vi "Actor Core.vi"(8 "error in":errorcluster caption="错误输入", 11 "P3AT in":refnum<class "RemoteP3AT.lvclass"> caption="操作者输入") -> (0 "error out":errorcluster caption="错误输出", 3 "Actor out":refnum<class "Actor.lvclass"> caption="操作者输出")   [LabVIEW 2014, in "RemoteP3AT.lvlib" / "RemoteP3AT.lvclass"]
doc: "(<B>文件名</B>：Actor Framework.lvlib:Actor.lvclass:Actor Core.vi)\n\n接收发送至操作者的消息，响应消息并处理可能导致操作者关闭的错误。\n\n子孙类重写该VI，使操作者完成特定的任务。使用调用父方法节点实现重写。"
uses:
  RemoteP3AT.lvclass
  <vilib>/ActorFramework/Actor/Actor.lvclass
  ctl/Point.ctl
  ctl/P3AT_Panel.ctl
  <userlib>/ROS for LabVIEW Software/ROS/Code/Console/Servers/ServerSubs/TopicDef.ctl
  <userlib>/ROS for LabVIEW Software/ROS/Code/SubVIs/_ROSDirection.ctl
  RemoteP3AT.lvclass/RemoteP3AT.ctl
  <vilib>/ActorFramework/Actor/Actor.lvclass/Actor.ctl
  <vilib>/ActorFramework/Message Enqueuer/Message Enqueuer.lvclass/Message Enqueuer.ctl
  <vilib>/ActorFramework/Message Enqueuer/Enqueue.vi
  Global_var/Global_var.vi
  <vilib>/ActorFramework/Message Priority Queue/Priority Enqueue.vi
  Wrapper_lib/zsActor/ActorWrapper.lvclass
panel:
  out "P3AT_Ini_Pose":T1
  out "P3AT_Panel":T2={"max_vel"=0.49056603773584906, "max_rot"=0.5094339622641509, "Control_Mode"=enum."Joy"} {"max_rot" scale=0.0..1.0; "max_vel" scale=0.0..1.0}
  out "vel_cal":cluster{"rot_z":dbl, "lin_x":dbl}
  out "local_goal":T3
  in  "停止信号":bool
  # "P3AT_Panel 此处不起作用"
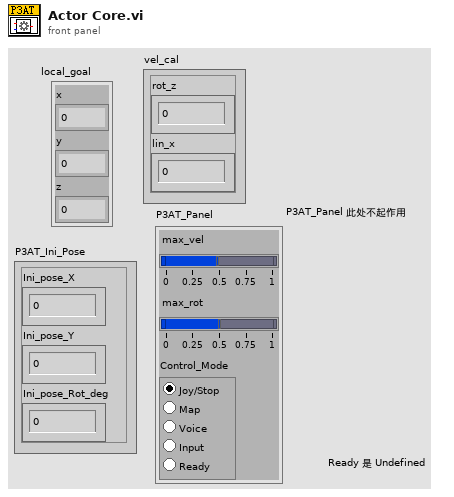
[diagram p1: front panel]
types:
  T1 = cluster{"Ini_pose_X":dbl, "Ini_pose_Y":dbl, "Ini_pose_Rot_deg":dbl}
  T2 = typedef "P3AT_Panel.ctl" = cluster{"max_vel":dbl, "max_rot":dbl, "Control_Mode":enum32{"Joy", "Map", "Voice", "Input", "Undefined"}}
  T3 = typedef "Point.ctl" = cluster{"x":dbl, "y":dbl, "z":dbl}
  T4 = typedef "TopicDef.ctl" = cluster{"Topic":string, "Type":string, "Action":T5, "Update (ms)":u16, "queue size":u16}
  T5 = typedef "_ROSDirection.ctl" = enum16{"Node", "Publisher", "Subscriber", "ServiceClient", "ServiceProvider"}
  T6 = typedef "_ROSControl.ctl" = cluster{"topic port":u16, "Node":string, "topic":string, "type":string, "node port":u16, "error ":errorcluster, "Direction":T5, "Update (ms)":u16, "FIFO size":u16}
  T7 = enum32{"Joy", "Map", "Voice", "Input", "Undefined"}
  T8 = typedef "P3AT_Current.ctl" = cluster{"max_vel":dbl, "max_rot":dbl, "now_pose_X":dbl, "now_pose_Y":dbl, "now_pose_Rot_deg":dbl, "Control_Mode":enum32{"Joy", "Map", "Voice", "Input", "Undefined"}}
  T9 = cluster{"now_pose_X":dbl, "now_pose_Y":dbl, "now_pose_Rot_deg":dbl}
  T10 = typedef "Robot_Position.ctl" = cluster{"global x":dbl, "global y":dbl, "global z":dbl, "global_rot":dbl, " floor NO.":dbl}
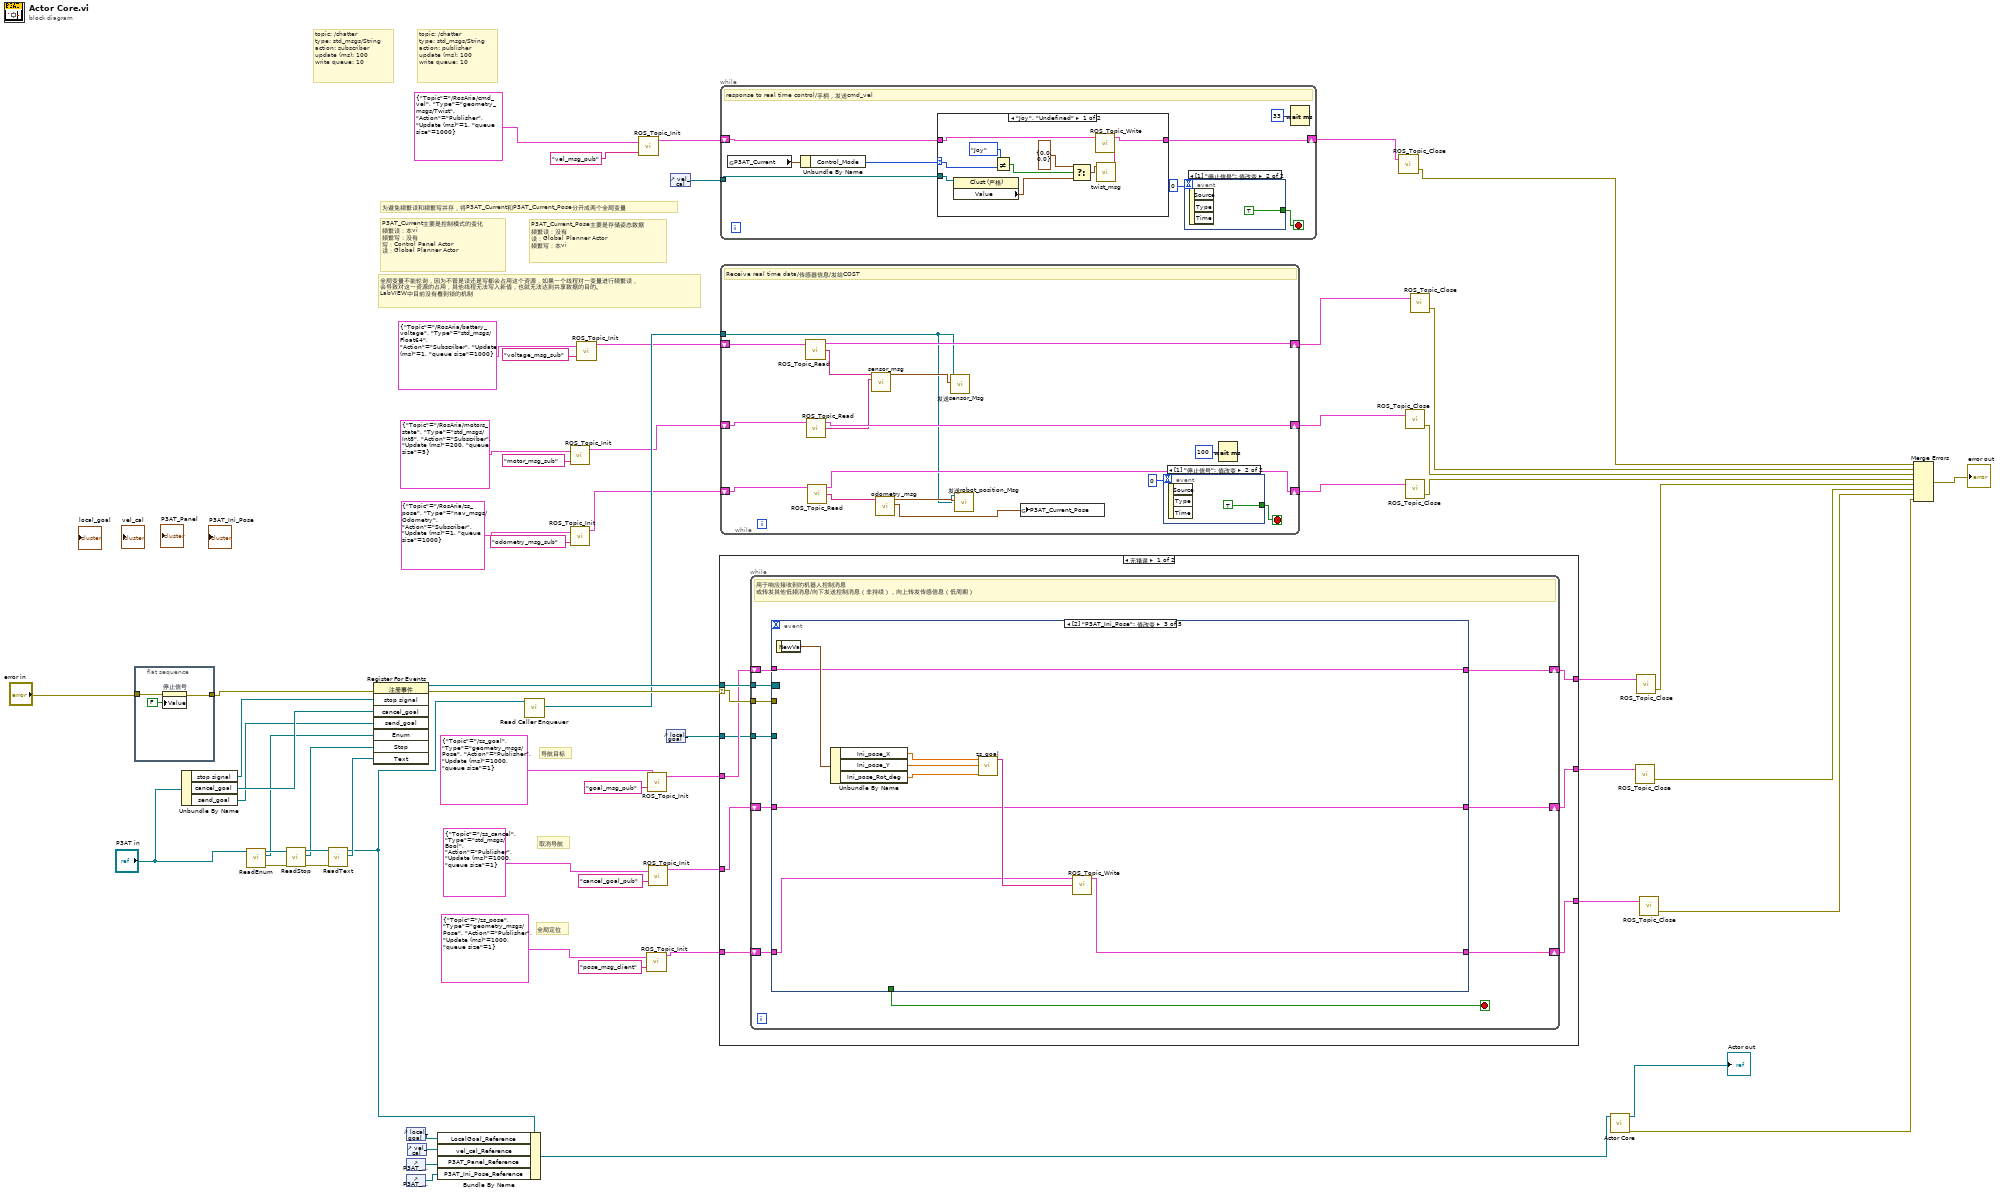
[diagram p0: block diagram]
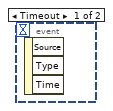
[diagram p3: hidden frame]
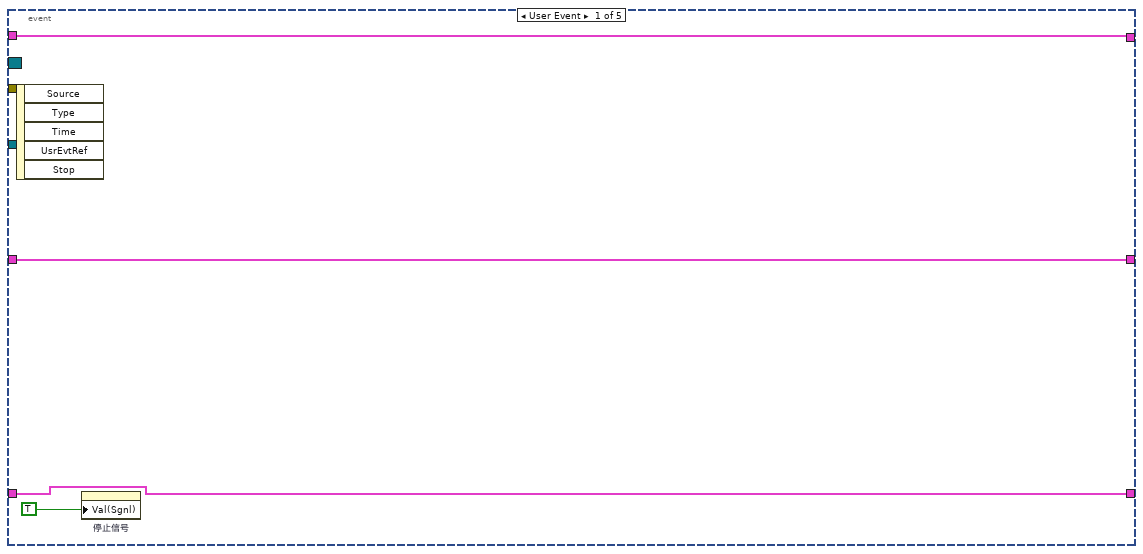
[diagram p4: hidden frame]
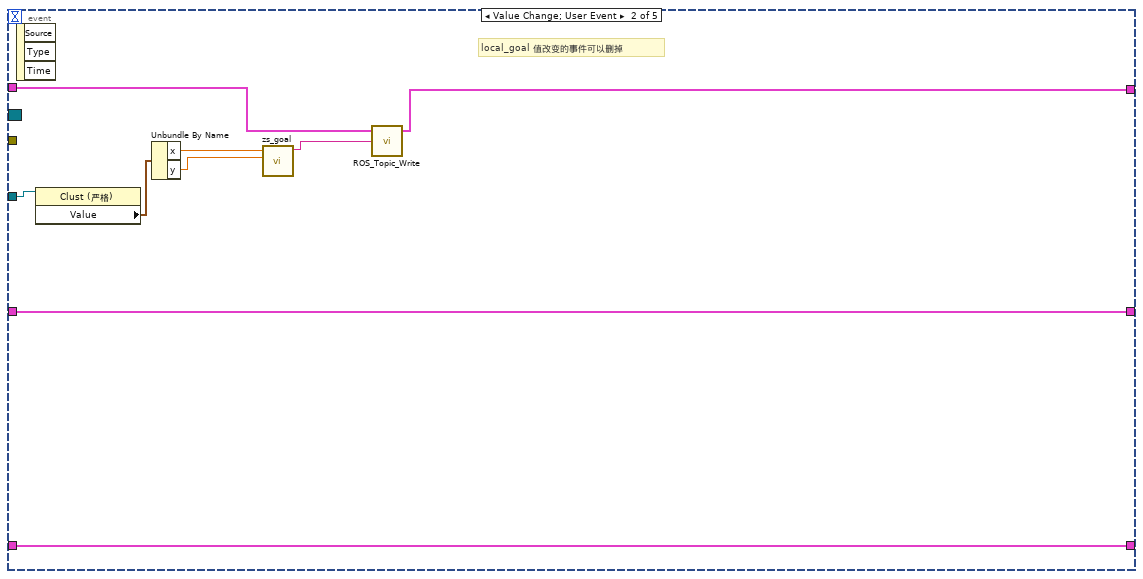
[diagram p5: hidden frame]
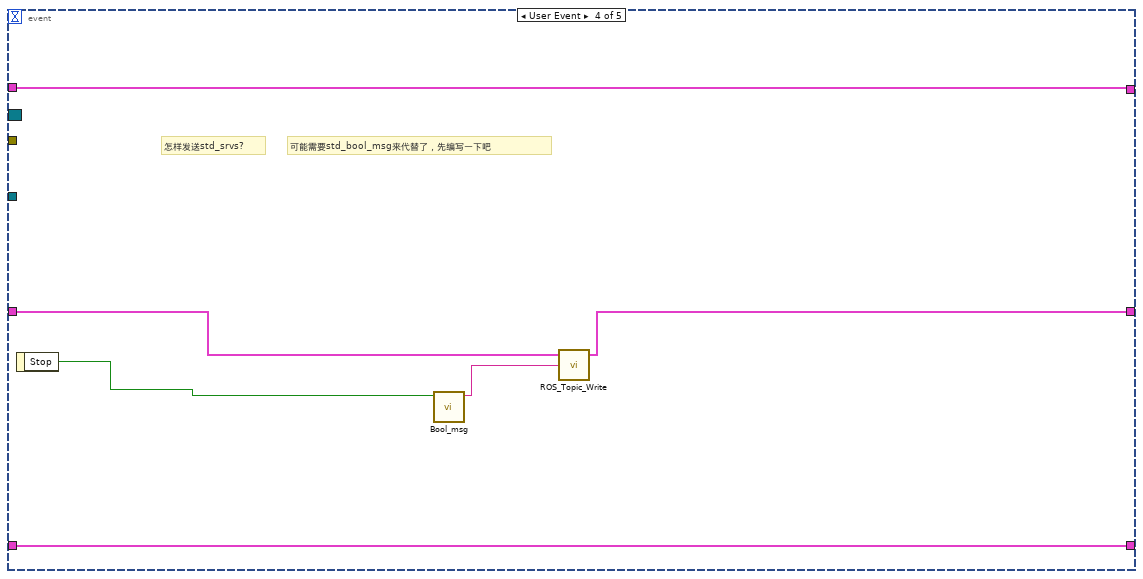
[diagram p6: hidden frame]
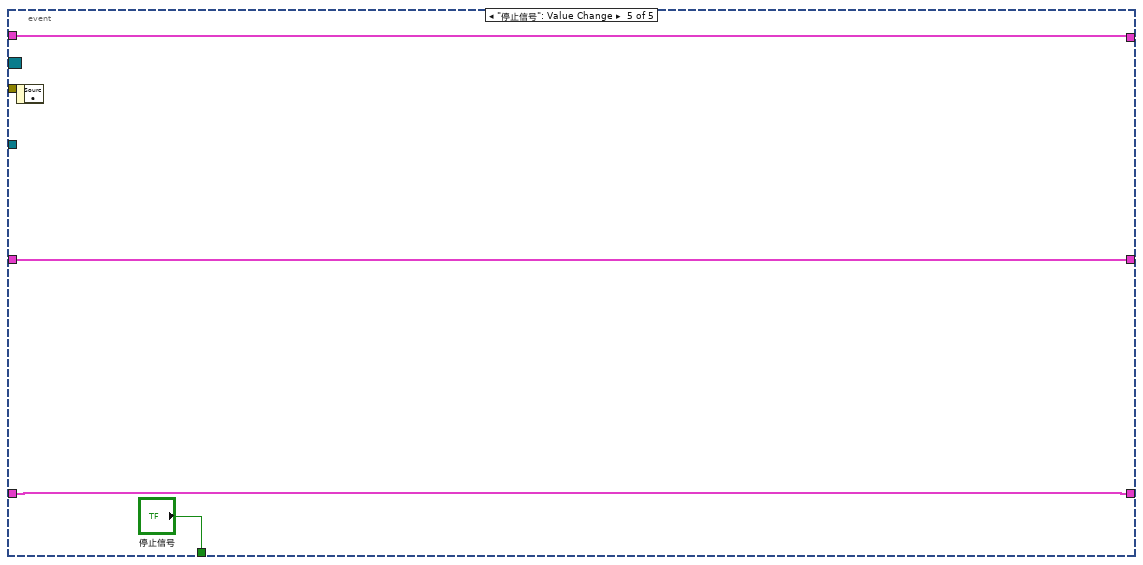
[diagram p7: hidden frame]
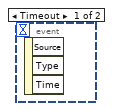
[diagram p9: hidden frame]
diagram:
  # "全局变量不能轮询，因为不管是读还是写都会占用这个资源，如果一个线程对一变量进行频繁读，\n会导致对这一资源的占用，其他线程无法写入新值，也就无法达到共享数据的目的。\nLabVIEW中目前没有看到锁的机制"
  # "全局定位"
  # "P3AT_Current_Pose主要是存储姿态数据\n频繁读：没有\n读：Global Planner Actor\n频繁写：本vi"
  # "P3AT_Current主要是控制模式的变化\n频繁读：本vi\n频繁写：没有\n写：Control Panel Actor\n读：Global Planner Actor"
  # "为避免频繁读和频繁写并存，将P3AT_Current和P3AT_Current_Pose分开成两个全局变量"
  # "导航目标"
  # "取消导航"
  # "topic: /chatter\ntype: std_msgs/String\naction: subscriber\nupdate (ms): 100\nwrite queue: 10"
  # "topic: /chatter\ntype: std_msgs/String\naction: publisher\nupdate (ms): 100\nwrite queue: 10"
  n1 = flat-sequence {
    tunnel: [w64] -> w58
    tunnel: "error in" -> [w63]
    frame #0 {
      n2 = property on="停止信号" class="Bool (严格)"(error in=w63, "Value"=FALSE ("停止信号")) -> (error out=w64:errorcluster)  [unwired: 1 in, 1 out]
    }
  }
  n3 = Unbundle By Name("P3AT in") -> ("stop signal"=w57:refnum<user-event>, "cancel_goal"=w56:refnum<user-event>, "send_goal"=w1:refnum<user-event>)
  n4 = call-dynamic "ReadEnum.vi"("zsActor输入"="P3AT in") -> ("error out"=w53:errorcluster, "Enum"=w50:refnum<user-event>, "zsActor输出"=w55:refnum<class "RemoteP3AT.lvclass">)  [unwired: 8 in]
  n5 = call-dynamic "ReadStop.vi"("error in (no error)"=w53, "zsActor输入"=w55) -> ("error out"=w52:errorcluster, "Stop"=w49:refnum<user-event>, "zsActor输出"=w54:refnum<class "RemoteP3AT.lvclass">)  [unwired: 7 in]
  n6 = call-dynamic "ReadText.vi"("error in (no error)"=w52, "zsActor输入"=w54) -> ("Text"=w48:refnum<user-event>, "zsActor输出"=w19:refnum<class "RemoteP3AT.lvclass">)  [unwired: 7 in, 1 out]
  n7 = register-events(error in=w58, w57, w56, w1, w50, w49, w48) -> (reference out=w60:refnum<event-registration>, error out=w61:errorcluster)  [unwired: 1 in]
  n8 = control-ref of="P3AT_Panel"() -> (w10:refnum<vi>)
  n9 = control-ref of="local_goal"() -> (w17:refnum<vi>)
  n10 = control-ref of="P3AT_Ini_Pose"() -> (w3:refnum<vi>)
  n11 = control-ref of="vel_cal"() -> (w12:refnum<vi>)
  n12 = Bundle By Name(cluster=w19, "LocalGoal_Reference"=w17, "vel_cal_Reference"=w12, "P3AT_Panel_Reference"=w10, "P3AT_Ini_Pose_Reference"=w3) -> (w18:refnum<class "RemoteP3AT.lvclass">)
  n13 = call <vilib>:"Read Caller Enqueuer.vi"("Actor"=w19) -> ("Caller Enqueuer"=w47:refnum<class "Message Enqueuer.lvclass">)  [unwired: 10 in]
  n14 = call <userlib>:"ROS_Topic_Init.vi"("Definitions"=T4 {"Topic"="/RosAria/motors_state", "Type"="std_msgs/Int8", "Action"=enum."Subscriber", "Update (ms)"=200, "queue size"=5}, "node"="motor_msg_sub") -> ("ROS out"=w28:T6)  [unwired: 1 in, 1 out]
  n15 = call <userlib>:"ROS_Topic_Init.vi"("Definitions"=T4 {"Topic"="/RosAria/zs_pose", "Type"="nav_msgs/Odometry", "Action"=enum."Subscriber", "Update (ms)"=1, "queue size"=1000}, "node"="odometry_msg_sub") -> ("ROS out"=w24:T6)  [unwired: 1 in, 1 out]
  n16 = call <userlib>:"ROS_Topic_Init.vi"("Definitions"=T4 {"Topic"="/RosAria/battery_voltage", "Type"="std_msgs/Float64", "Action"=enum."Subscriber", "Update (ms)"=1, "queue size"=1000}, "node"="voltage_msg_sub") -> ("ROS out"=w30:T6)  [unwired: 1 in, 1 out]
  n17 = call <userlib>:"ROS_Topic_Init.vi"("Definitions"=T4 {"Topic"="/RosAria/cmd_vel", "Type"="geometry_msgs/Twist", "Action"=enum."Publisher", "Update (ms)"=1, "queue size"=1000}, "node"="vel_msg_pub") -> ("ROS out"=w31:T6)  [unwired: 1 in, 1 out]
  n18 = call <userlib>:"ROS_Topic_Init.vi"("Definitions"=T4 {"Topic"="/zs_pose", "Type"="geometry_msgs/Pose", "Action"=enum."Publisher", "Update (ms)"=1000, "queue size"=1}, "node"="pose_msg_client") -> ("ROS out"=w4:T6)  [unwired: 1 in, 1 out]
  n19 = call <userlib>:"ROS_Topic_Init.vi"("Definitions"=T4 {"Topic"="/zs_goal", "Type"="geometry_msgs/Pose", "Action"=enum."Publisher", "Update (ms)"=1000, "queue size"=1}, "node"="goal_msg_pub") -> ("ROS out"=w16:T6)  [unwired: 1 in, 1 out]
  n20 = call <userlib>:"ROS_Topic_Init.vi"("Definitions"=T4 {"Topic"="/zs_cancel", "Type"="std_msgs/Bool", "Action"=enum."Publisher", "Update (ms)"=1000, "queue size"=1}, "node"="cancel_goal_pub") -> ("ROS out"=w15:T6)  [unwired: 1 in, 1 out]
  n21 = control-ref of="local_goal"() -> (w9:refnum<vi>)
  n22 = control-ref of="vel_cal"() -> (w11:refnum<vi>)
  n23 = case shown="无错误" w61 {
    selector: w61 -> [w73 _]
    tunnel: w60 -> [w74 _]
    tunnel: w16 -> [w72 w119]
    tunnel: w15 -> [w71 w118]
    tunnel: [w70 w119] -> w14
    tunnel: [w69 w118] -> w13
    tunnel: w9 -> [w68 _]
    tunnel: w4 -> [w67 w117]
    tunnel: [w66 w117] -> w2
    frame No Error {
      n24 = while {
        tunnel: w74 -> [w84]
        tunnel: w73 -> [w82]
        shift-right: [w81] -> w70
        shift-left: w72 -> [w80]
        shift-right: [w78] -> w69
        shift-left: w71 -> [w79]
        tunnel: w68 -> [w77]
        shift-right: [w75] -> w66
        shift-left: w67 -> [w76]
        stop <- w83 stop-if-true
        # "用于响应接收到的机器人控制消息\n或转发其他低频消息/向下发送控制消息（非持续），向上转发传感信息（低周期）"
        n25 = event shown="[2] \"P3AT_Ini_Pose\": 值改变" {
          selector: w84 -> [_ _ _ _ _]
          dyn-events: _ -> [_ _ _ _ _]
          timeout: _ -> [_ _ _ _ _]
          tunnel: [_ _ _ _ "停止信号"] -> w83
          tunnel: w82 -> [_ _ _ _ _]
          tunnel: w80 -> [w87 w95 w98 w110 w115]
          tunnel: [w87 w93 w98 w110 w115] -> w81
          tunnel: w79 -> [w86 w92 w99 w112 w114]
          tunnel: [w86 w92 w99 w111 w114] -> w78
          tunnel: w77 -> [_ w91 _ _ _]
          tunnel: w76 -> [w85 w89 w101 w109 w113]
          tunnel: [w85 w89 w100 w109 w113] -> w75
          event User Event {
            n26 = event-data() -> ()  [unwired: 1 in, 5 out]
            n27 = property on="停止信号" class="Bool (严格)"("Val(Sgnl)"=TRUE ("值(信号)")) -> ()  [unwired: 2 in, 2 out]
          }
          event Value Change; User Event {
            # "local_goal 值改变的事件可以删掉"
            n28 = event-data() -> ()  [unwired: 1 in, 3 out]
            n29 = property class="Clust (严格)"(reference=w91) -> ("Value"=w90:T3)  [unwired: 1 in, 2 out]
            n30 = Unbundle By Name(w90) -> ("x"=w97:dbl, "y"=w96:dbl)
            n31 = call "zs_goal.vi"("Point.y"=w96, "Point.x"=w97) -> ("msg out"=w94:string)  [unwired: 9 in]
            n32 = call <userlib>:"ROS_Topic_Write.vi"("Msg in"=w94, "ROS in"=w95) -> ("ROS out"=w93:T6)  [unwired: 2 in, 1 out]
          }
          event "P3AT_Ini_Pose": Value Change {
            n33 = event-data() -> ("NewVal"=w106:T1)  [unwired: 1 in]
            n34 = Unbundle By Name(w106) -> ("Ini_pose_X"=w105:dbl, "Ini_pose_Y"=w104:dbl, "Ini_pose_Rot_deg"=w103:dbl)
            n35 = call "zs_goal.vi"("Yaw (z)"=w103, "Point.y"=w104, "Point.x"=w105) -> ("msg out"=w102:string)  [unwired: 8 in]
            n36 = call <userlib>:"ROS_Topic_Write.vi"("Msg in"=w102, "ROS in"=w101) -> ("ROS out"=w100:T6)  [unwired: 2 in, 1 out]
          }
          event User Event {
            # "可能需要std_bool_msg来代替了，先编写一下吧"
            # "怎样发送std_srvs?"
            n37 = event-data() -> ("Stop"=w107:bool)  [unwired: 1 in]
            n38 = call "Bool_msg.vi"("Boolean"=w107) -> ("msg out"=w108:string)  [unwired: 10 in]
            n39 = call <userlib>:"ROS_Topic_Write.vi"("Msg in"=w108, "ROS in"=w112) -> ("ROS out"=w111:T6)  [unwired: 2 in, 1 out]
          }
          event "停止信号": Value Change {
            n40 = event-data() -> ()  [unwired: 1 in, 1 out]
          }
        }
      }
    }
    frame Error {
    }
  }
  n41 = while {
    shift-right: [w123] -> w32
    shift-left: w31 -> [w124]
    tunnel: w11 -> [w122]
    stop <- w126 stop-if-true
    # "response to real time control/手柄，发送cmd_vel"
    n42 = global read "Global_var.vi" "P3AT_Current"() -> (w120:T8)
    n43 = Unbundle By Name(w120) -> ("Control_Mode"=w121:T7)
    n44 = case shown="\"Joy\", \"Undefined\"" w121 {
      selector: w121 -> [w132 _]
      tunnel: w124 -> [w137 w138]
      tunnel: [w136 w138] -> w123
      tunnel: w122 -> [w135 _]
      frame "Joy", "Undefined" {
        n45 = property class="Clust (严格)"(reference=w135) -> ("Value"=w130:cluster{"rot_z":dbl, "lin_x":dbl})  [unwired: 1 in, 2 out]
        n46 = Not Equal?(x=T7."Joy" ("Control_Mode"), y=w132) -> (x != y?=w131:bool)
        n47 = Select(t=cluster{"rot_z":dbl, "lin_x":dbl} {"rot_z"=0.0, "lin_x"=0.0} ("值"), s=w131, f=w130) -> (s? t:f=w128:cluster{"rot_z":dbl, "lin_x":dbl})
        n48 = call "twist_msg.vi"("vel_cal"=w128) -> ("msg out"=w134:string)  [unwired: 10 in]
        n49 = call <userlib>:"ROS_Topic_Write.vi"("Msg in"=w134, "ROS in"=w137) -> ("ROS out"=w136:T6)  [unwired: 2 in, 1 out]
      }
      frame "Map".."Input", Default {
      }
    }
    n50 = event shown="[1] \"停止信号\": 值改变" {
      selector: _ -> [_ _]
      dyn-events: _ -> [_ _]
      timeout: 0 -> [_ _]
      tunnel: [_ TRUE] -> w126
      event Timeout {
        n51 = event-data() -> ()  [unwired: 1 in, 3 out]
      }
      event "停止信号": Value Change {
        n52 = event-data() -> ()  [unwired: 1 in, 3 out]
      }
    }
    n53 = Wait (ms)(milliseconds to wait=u32 33 ("等待时间（毫秒）")) -> ()  [unwired: 1 out]
  }
  n54 = while {
    tunnel: w47 -> [w141]
    shift-right: [w151] -> w29
    shift-left: w30 -> [w152]
    shift-right: [w149] -> w27
    shift-left: w28 -> [w150]
    shift-right: [w147] -> w23
    shift-left: w24 -> [w148]
    stop <- w154 stop-if-true
    # "Receive real time data/传感器信息/发给COST"
    n55 = call <userlib>:"ROS_Topic_Read.vi"("ROS in"=w152) -> ("Reply"=w146:string, "ROS out"=w151:T6)  [unwired: 2 in, 1 out]
    n56 = call <userlib>:"ROS_Topic_Read.vi"("ROS in"=w150) -> ("Reply"=w145:string, "ROS out"=w149:T6)  [unwired: 2 in, 1 out]
    n57 = call <userlib>:"ROS_Topic_Read.vi"("ROS in"=w148) -> ("Reply"=w144:string, "ROS out"=w147:T6)  [unwired: 2 in, 1 out]
    n58 = call "sensor_msg.vi"("motor_msg in"=w145, "voltage_msg in"=w146) -> ("sensor_msg_cluster"=w143:cluster{"voltage":dbl, "motor":i8})  [unwired: 9 in]
    n59 = call "odometry_msg.vi"("odometry_msg in"=w144) -> ("Current_Pose"=w140:T9, "robot_position_cluster"=w142:T10)  [unwired: 9 in]
    n60 = call "发送sensor_Msg.vi"("值(信号)"=w143, "消息待入队列"=w141) -> ()  [unwired: 8 in, 2 out]
    n61 = call "发送robot_position_Msg.vi"("值(信号)"=w142, "消息待入队列"=w141) -> ()  [unwired: 8 in, 2 out]
    n62 = global write "Global_var.vi" "P3AT_Current_Pose"(w140) -> ()
    n63 = event shown="[1] \"停止信号\": 值改变" {
      selector: _ -> [_ _]
      dyn-events: _ -> [_ _]
      timeout: 0 -> [_ _]
      tunnel: [_ TRUE] -> w154
      event Timeout {
        n64 = event-data() -> ()  [unwired: 1 in, 3 out]
      }
      event "停止信号": Value Change {
        n65 = event-data() -> ()  [unwired: 1 in, 3 out]
      }
    }
    n66 = Wait (ms)(milliseconds to wait=u32 100 ("等待时间（毫秒）")) -> ()  [unwired: 1 out]
  }
  n67 = call <userlib>:"ROS_Topic_Close.vi"("ROS in"=w32) -> ("error out"=w33:errorcluster)  [unwired: 3 in]
  n68 = call <userlib>:"ROS_Topic_Close.vi"("ROS in"=w27) -> ("error out"=w35:errorcluster)  [unwired: 3 in]
  n69 = call <userlib>:"ROS_Topic_Close.vi"("ROS in"=w23) -> ("error out"=w20:errorcluster)  [unwired: 3 in]
  n70 = call <userlib>:"ROS_Topic_Close.vi"("ROS in"=w29) -> ("error out"=w34:errorcluster)  [unwired: 3 in]
  n71 = call-parent "Actor Core.vi"("Actor in"=w18) -> ("error out"=w6:errorcluster, "Actor out"=→"Actor out":refnum<class "Actor.lvclass">)  [unwired: 9 in]
  n72 = call <userlib>:"ROS_Topic_Close.vi"("ROS in"=w13) -> ("error out"=w22:errorcluster)  [unwired: 3 in]
  n73 = call <userlib>:"ROS_Topic_Close.vi"("ROS in"=w14) -> ("error out"=w21:errorcluster)  [unwired: 3 in]
  n74 = call <userlib>:"ROS_Topic_Close.vi"("ROS in"=w2) -> ("error out"=w5:errorcluster)  [unwired: 3 in]
  n75 = Merge Errors(w33, w34, w35, w20, w21, w22, w5, w6) -> (→"error out":errorcluster)
